vi "Publish.vi"(6 "connMeta":T1, 8 "error in (no error)":errorcluster, 9 "value":string, 10 "topic":string, 11 "mqtt in":refnum<class "MQTT Client.lvclass">) -> (0 "error out":errorcluster, 3 "mqtt out":refnum<class "MQTT Client.lvclass">)   [LabVIEW 2020, in "MQTT Client.lvclass"]
uses:
  MQTT Client.lvclass
  mqttTypedef/ConnectionMeta.ctl
  mqttTypedef/QosLevel.ctl
  mqttCmd/mqttCmdPublish/PublishMqttMsg.lvclass
  C:/Projects/Libraries/Gore SM 2020/mqtt-LabVIEW/src/class/mqtt/mqttCmd/BaseMqttMsg.lvclass
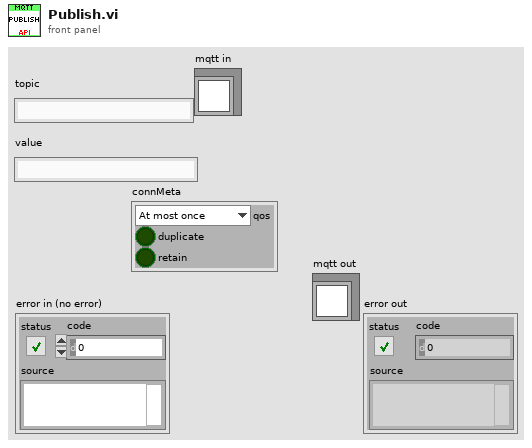
[diagram p1: front panel]
types:
  T1 = typedef "MQTT Client.lvclass/ConnectionMeta.ctl" = cluster{"qos":T2, "duplicate":bool, "retain":bool}
  T2 = typedef "MQTT Client.lvclass/QosLevel.ctl" = enum8{"At most once", "At least once", "Exactly once", "Reserved"}
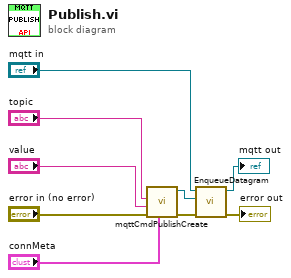
[diagram p0: block diagram]
diagram:
  n1 = call "mqttCmdPublishCreate.vi"("connMeta"="connMeta", "error in (no error)"="error in (no error)", "value"="value", "topic"="topic") -> ("error out"=w5:errorcluster, "mqttCmdPublish out"=w4:refnum<class "PublishMqttMsg.lvclass">)  [unwired: 6 in]
  n2 = call "EnqueueDatagram.vi"("error in (no error)"=w5, "mqttCmd"=w4, "mqtt in"="mqtt in") -> ("error out"=→"error out":errorcluster, "mqtt out"=→"mqtt out":refnum<class "MQTT Client.lvclass">)  [unwired: 7 in]
